vi "SetTitle.vi"(8 "error in (no error)":errorcluster, 10 "Title":string, 11 "reference in":refnum<class "TestView_Base.lvclass">) -> (0 "error out":errorcluster, 3 "reference in":refnum<class "TestView_Base.lvclass">)   [LabVIEW 2022 SP3, in "TestView_Base.lvlib" / "TestView_Base.lvclass"]
uses:
  TestView_Base.lvclass
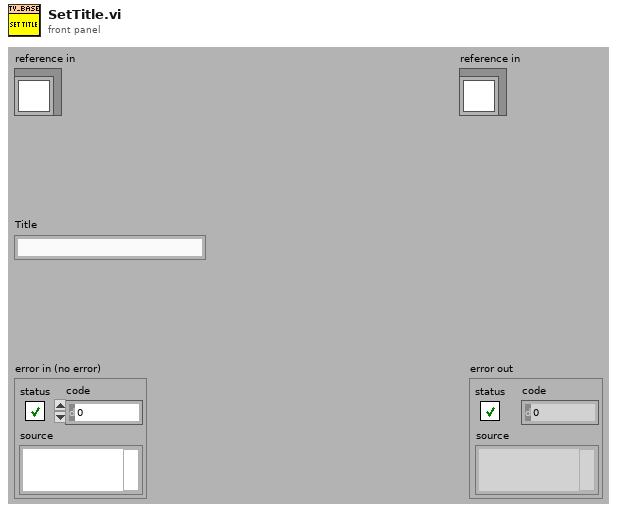
[diagram p1: front panel]
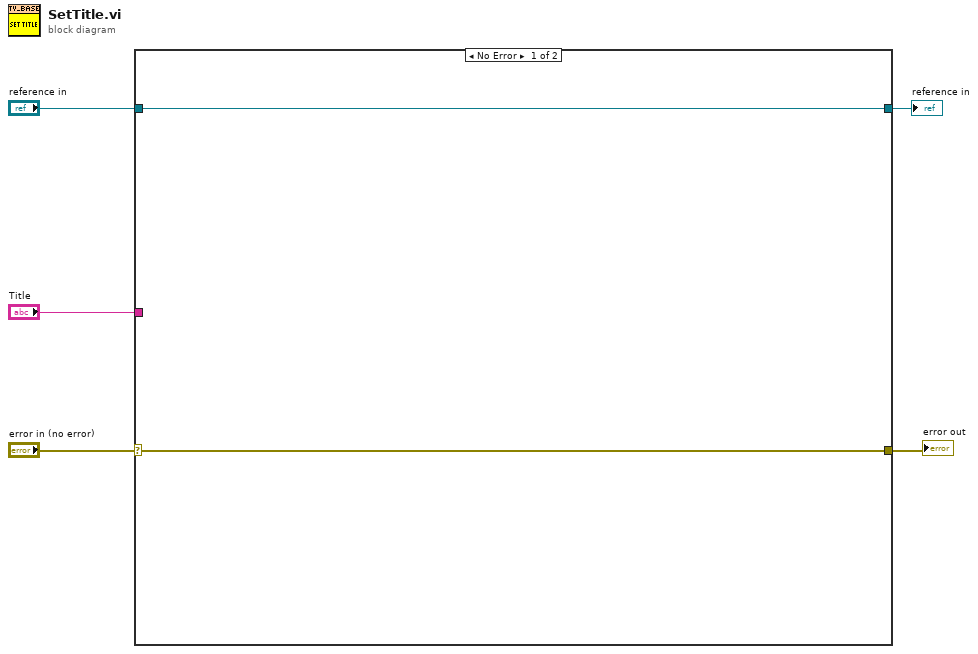
[diagram p0: block diagram]
diagram:
  n1 = case shown="No Error" "error in (no error)" {
    selector: "error in (no error)" -> [w6 w9]
    tunnel: [w6 w9] -> w4
    tunnel: [w7 w8] -> w2
    tunnel: "reference in" -> [w7 w8]
    tunnel: "Title" -> [_ _]
    frame No Error {
    }
    frame Error {
    }
  }
  "error out" <- w4
  "reference in" <- w2
